vi "grSim_Replacement Encoder.vi"(8 "error in (no error)":errorcluster, 10 "grSIM replacement":T1, 11 "Communication in":refnum<class "Communication.lvclass">) -> (0 "error out":errorcluster, 2 "robotControl":u8[](array[numeric]), 3 "Communication out":refnum<class "Communication.lvclass">)   [LabVIEW 2023, in "Communication.lvclass"]
uses:
  Communication.lvclass
  Controls/grSimReplacement.ctl
  Paths/grSim Packet Command UDP Test Folder/grSim/grSim RobotReplacement.ctl
  Paths/grSim Packet Command UDP Test Folder/grSim/grSim_BallReplacement.ctl
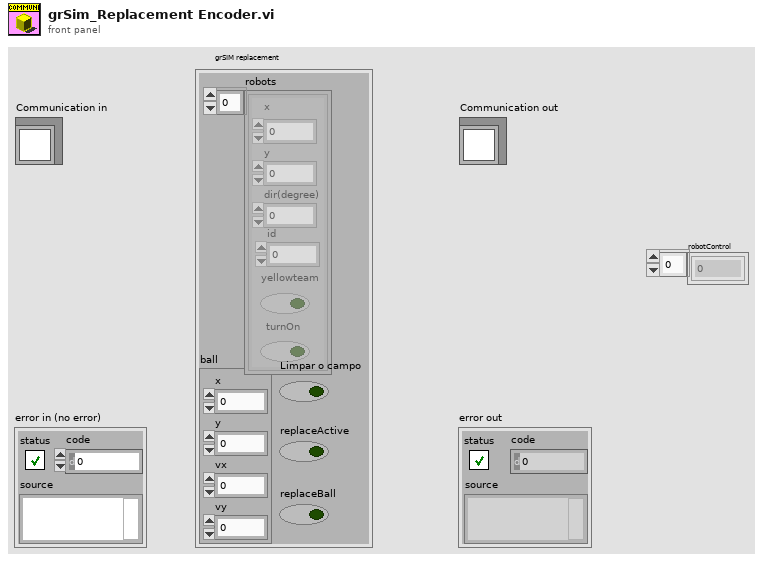
[diagram p1: front panel]
types:
  T1 = typedef "grSimReplacement.ctl" = cluster{"robots":T2[], "ball":T3, "replaceBall":bool, "replaceActive":bool, "Limpar o campo":bool}
  T2 = typedef "grSim RobotReplacement.ctl" = cluster{"x":dbl, "y":dbl, "dir(degree)":dbl, "yellowteam":bool, "id":u32, "turnOn":bool}
  T3 = typedef "grSim_BallReplacement.ctl" = cluster{"x":dbl, "y":dbl, "vx":dbl, "vy":dbl}
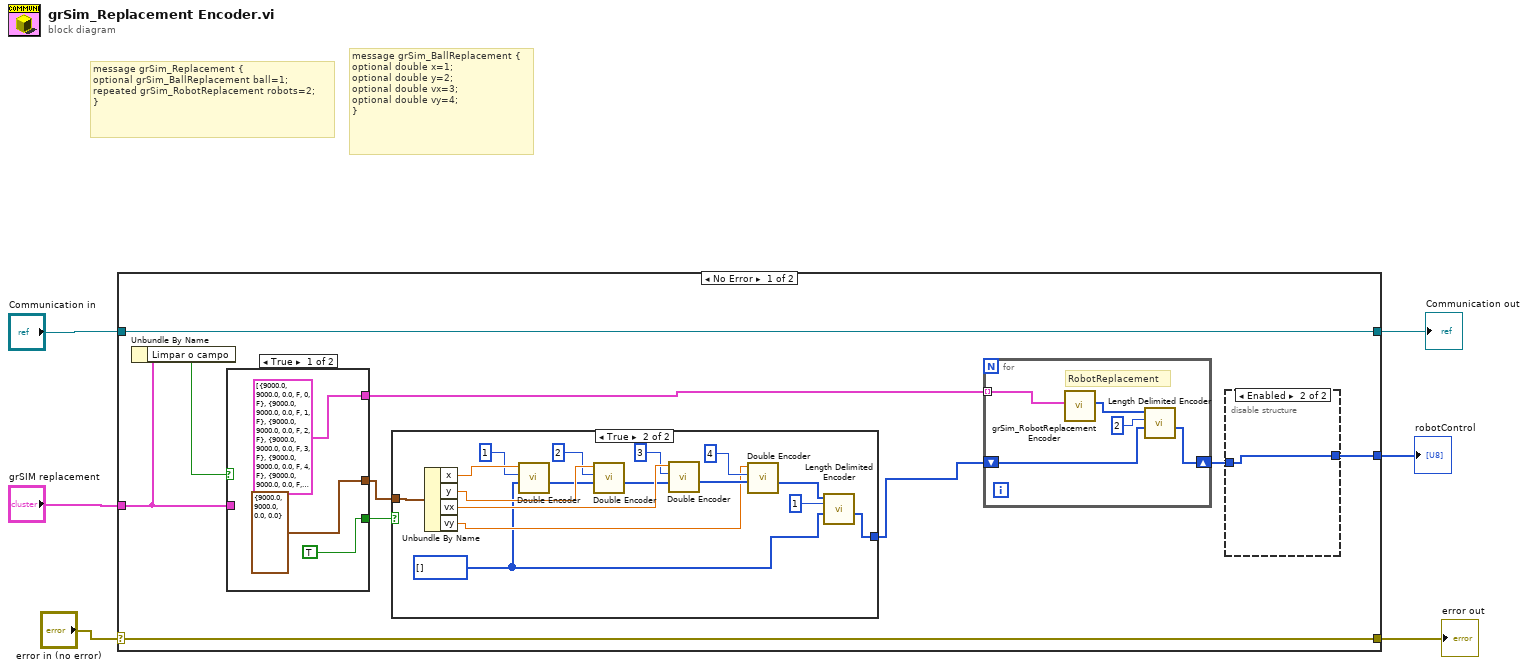
[diagram p0: block diagram]
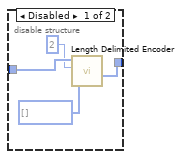
[diagram p2: hidden frame]
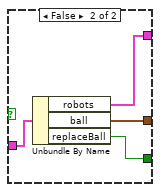
[diagram p3: hidden frame]
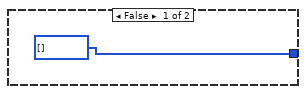
[diagram p4: hidden frame]
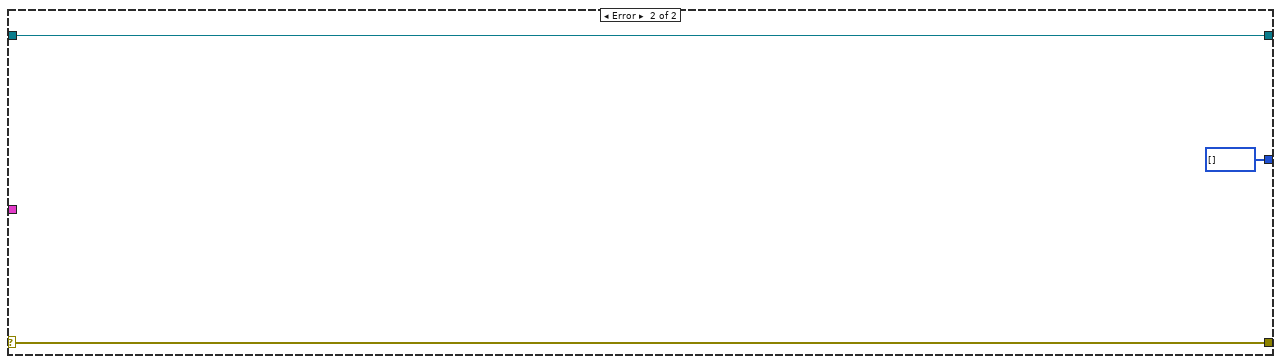
[diagram p5: hidden frame]
diagram:
  # "message grSim_Replacement {\noptional grSim_BallReplacement ball=1;\nrepeated grSim_RobotReplacement robots=2;\n}"
  # "message grSim_BallReplacement {\noptional double x=1;\noptional double y=2;\noptional double vx=3;\noptional double vy=4;\n}"
  n1 = case shown="No Error" "error in (no error)" {
    selector: "error in (no error)" -> [w15 w53]
    tunnel: [w15 w53] -> w5
    tunnel: [w16 w52] -> w3
    tunnel: "Communication in" -> [w16 w52]
    tunnel: "grSIM replacement" -> [w8 _]
    tunnel: [w9 u8[] [] ("Array")] -> w1
    frame No Error {
      n2 = Unbundle By Name(w8) -> ("Limpar o campo"=w7:bool)
      n3 = case shown="True" w7 {
        tunnel: w8 -> [_ w25]
        tunnel: [TRUE w28] -> w14
        tunnel: [T3 {"x"=9000.0, "y"=9000.0, "vx"=0.0, "vy"=0.0} ("ball") w27] -> w13
        tunnel: [T2[] [{"x"=9000.0, "y"=9000.0, "dir(degree)"=0.0, "yellowteam"=FALSE, "id"=0, "turnOn"=FALSE}, {"x"=9000.0, "y"=9000.0, "dir(degree)"=0.0, "yellowteam"=FALSE, "id"=1, "turnOn"=FALSE}, {"x"=9000.0, "y"=9000.0, "dir(degree)"=0.0, "yellowteam"=FALSE, "id"=2, "turnOn"=FALSE}, {"x"=9000.0, "y"=9000.0, "dir(degree)"=0.0, "yellowteam"=FALSE, "id"=3, "turnOn"=FALSE}, {"x"=9000.0, "y"=9000.0, "dir(degree)"=0.0, "yellowteam"=FALSE, "id"=4, "turnOn"=FALSE}, {"x"=9000.0, "y"=9000.0, "dir(degree)"=0.0, "yellowteam"=FALSE, "id"=5, "turnOn"=FALSE}, {"x"=9000.0, "y"=9000.0, "dir(degree)"=0.0, "yellowteam"=TRUE, "id"=0, "turnOn"=FALSE}, {"x"=9000.0, "y"=9000.0, "dir(degree)"=0.0, "yellowteam"=TRUE, "id"=1, "turnOn"=FALSE}, {"x"=9000.0, "y"=9000.0, "dir(degree)"=0.0, "yellowteam"=TRUE, "id"=2, "turnOn"=FALSE}, {"x"=9000.0, "y"=9000.0, "dir(degree)"=0.0, "yellowteam"=TRUE, "id"=3, "turnOn"=FALSE}, {"x"=9000.0, "y"=9000.0, "dir(degree)"=0.0, "yellowteam"=TRUE, "id"=4, "turnOn"=FALSE}, {"x"=9000.0, "y"=9000.0, "dir(degree)"=0.0, "yellowteam"=TRUE, "id"=5, "turnOn"=FALSE}] ("robots") w26] -> w12
        frame True {
        }
        frame False {
          n4 = Unbundle By Name(w25) -> ("robots"=w26:T2[], "ball"=w27:T3, "replaceBall"=w28:bool)
        }
      }
      n5 = case shown="True" w14 {
        tunnel: w13 -> [_ w50]
        tunnel: [u8[] [] ("Array") w35] -> w10
        frame False {
        }
        frame True {
          w37 = u8[] [] ("Array")
          n6 = Unbundle By Name(w50) -> ("x"=w49:dbl, "y"=w48:dbl, "vx"=w47:dbl, "vy"=w39:dbl)
          n7 = call "Double Encoder.vi"("Array In"=w37, "Key"=1, "Value"=w49) -> ("Array"=w45:u8[])  [unwired: 8 in]
          n8 = call "Double Encoder.vi"("Array In"=w45, "Key"=2, "Value"=w48) -> ("Array"=w46:u8[])  [unwired: 8 in]
          n9 = call "Double Encoder.vi"("Array In"=w46, "Key"=3, "Value"=w47) -> ("Array"=w44:u8[])  [unwired: 8 in]
          n10 = call "Double Encoder.vi"("Array In"=w44, "Key"=4, "Value"=w39) -> ("Array"=w38:u8[])  [unwired: 8 in]
          n11 = call "Length Delimited Encoder.vi"("Original Array In"=w37, "Key"=1, "Array In to be added"=w38) -> ("Array"=w35:u8[])  [unwired: 8 in]
        }
      }
      n12 = for {
        shift-right: [w29] -> w11
        shift-left: w10 -> [w30]
        tunnel: w12 -> [w33] mode=indexing
        # "RobotReplacement"
        n13 = call "grSim_RobotReplacement Encoder.vi"("Robot"=w33) -> ("Array out"=w32:u8[])  [unwired: 10 in]
        n14 = call "Length Delimited Encoder.vi"("Original Array In"=w30, "Key"=2, "Array In to be added"=w32) -> ("Array"=w29:u8[])  [unwired: 8 in]
      }
      n15 = disable-structure shown="Enabled" {
        disable-tunnel: w11 -> [w20 w21]
        disable-tunnel: [w17 w21] -> w9
        frame Disabled {
          n16 = call "Length Delimited Encoder.vi"("Original Array In"=u8[] [] ("Array"), "Key"=2, "Array In to be added"=w20) -> ("Array"=w17:u8[])  [unwired: 8 in]
        }
        frame Enabled {
        }
      }
    }
    frame Error {
    }
  }
  "error out" <- w5
  "Communication out" <- w3
  "robotControl" <- w1
